vi "Set Internal Temp Limits.vi"(6 "parseError? T:Yes":bool=TRUE, 8 "error in (no error)":errorcluster, 9 "InternMin (-20.00 °C)":dbl=-20.0, 10 "InternMax (50.00 °C)":dbl=50.0, 11 "VISA resource name":refnum<visa-resource-name>) -> (0 "error out":errorcluster, 3 "VISA resource name out":refnum<visa-resource-name>)   [LabVIEW 2018, in "JULABO DeviceDriver.lvlib"]
doc: "This VI adjusts the upper and lower temperature limit for the internal temperature during external temperature control. <B>InternMax</B> and <B>InternMin</B> determine fixed limits for the temperature within the internal bath. The temperature controller cannot exceed these limits even if it would be necessary for achieving the temperature in an external system. Therefore it is possible that the external setpoint cannot be achieved.\n\nNote:\nThis function is not available for devices which do not have an external sensor plug. For these instruments the VI will return an error (-08 INVALID COMMAND)."
uses:
  JULABO DeviceDriver.lvlib
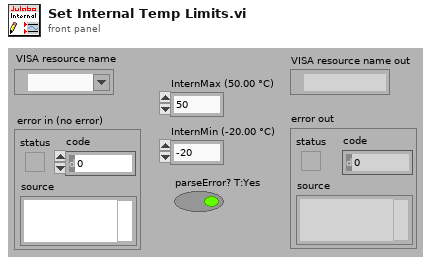
[diagram p1: front panel]
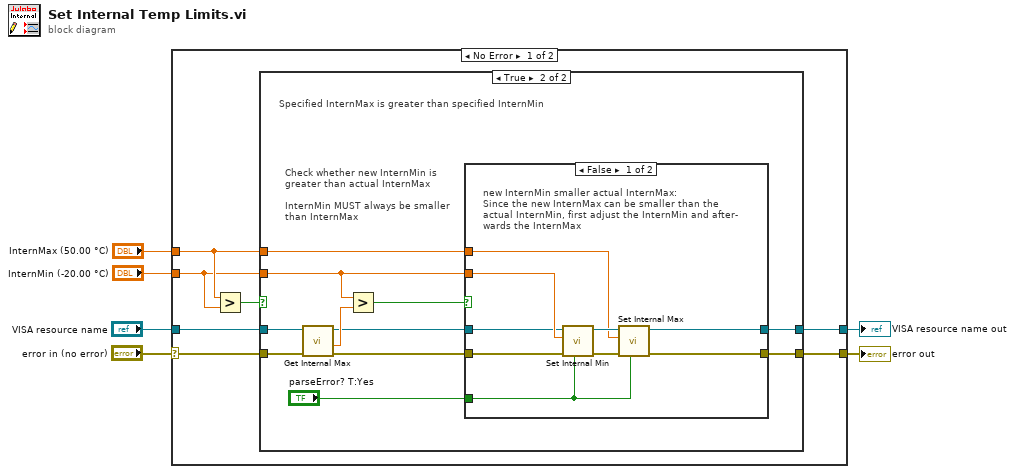
[diagram p0: block diagram]
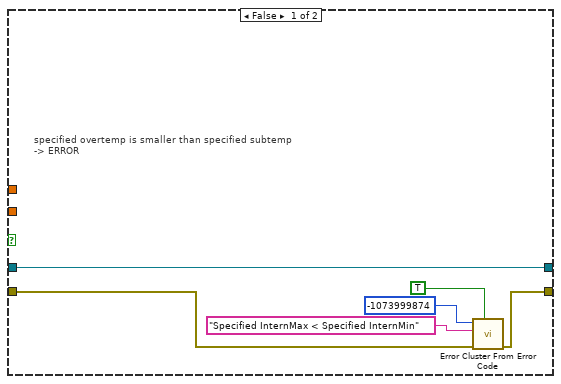
[diagram p2: hidden frame]
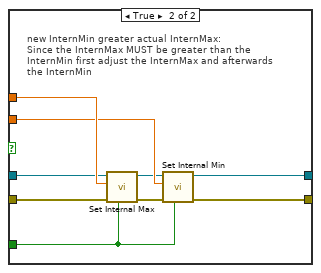
[diagram p3: hidden frame]
diagram:
  n1 = case shown="No Error" "error in (no error)" {
    selector: "error in (no error)" -> [w10 w49]
    tunnel: "VISA resource name" -> [w13 w50]
    tunnel: [w12 w50] -> w5
    tunnel: [w11 w49] -> w4
    tunnel: "InternMax (50.00 °C)" -> [w8 _]
    tunnel: "InternMin (-20.00 °C)" -> [w7 _]
    frame No Error {
      n2 = Greater?(x=w8, y=w7) -> (0:w9:bool)
      n3 = case shown="True" w9 {
        tunnel: w13 -> [w19 w26]
        tunnel: [w19 w29] -> w12
        tunnel: [w15 w28] -> w11
        tunnel: w10 -> [w14 w25]
        tunnel: w8 -> [_ w27]
        tunnel: w7 -> [_ w23]
        frame False {
          # "specified overtemp is smaller than specified subtemp\n-> ERROR"
          n4 = call <vilib>:"Error Cluster From Error Code.vi"("show call chain? (False)"=TRUE, "error in (no error)"=w14, "error message (\"\")"="Specified InternMax < Specified InternMin" ("error message (\"\")"), "error code (0)"=-1073999874) -> ("error out"=w15:errorcluster)  [unwired: 5 in]
        }
        frame True {
          # "Check whether new InternMin is\ngreater than actual InternMax\n\nInternMin MUST always be smaller\nthan InternMax"
          # "Specified InternMax is greater than specified InternMin"
          n5 = call "Get Internal Max.vi"("error in (no error)"=w25, "VISA resource name"=w26) -> ("error out"=w21:errorcluster, "IntMax (out)"=w24:dbl, "VISA resource name out"=w22:refnum<visa-resource-name>)  [unwired: 7 in]
          n6 = Greater?(x=w23, y=w24) -> (0:w20:bool)
          n7 = case shown="False" w20 {
            tunnel: "parseError? T:Yes" -> [w39 w48]
            tunnel: [w36 w41] -> w29
            tunnel: [w35 w40] -> w28
            tunnel: w27 -> [w34 w47]
            tunnel: w23 -> [w33 w46]
            tunnel: w22 -> [w32 w45]
            tunnel: w21 -> [w31 w44]
            frame False {
              # "new InternMin smaller actual InternMax:\nSince the new InternMax can be smaller than the \nactual InternMin, first adjust the InternMin and after-\nwards the InternMax"
              n8 = call "Set Internal Min.vi"("parseError? T:Yes"=w39, "error in (no error)"=w31, "InternMin (-20.00 °C)"=w33, "VISA resource name"=w32) -> ("error out"=w37:errorcluster, "VISA resource name out"=w38:refnum<visa-resource-name>)  [unwired: 6 in]
              n9 = call "Set Internal Max.vi"("parseError? T:Yes"=w39, "error in (no error)"=w37, "InternMax (50.00 °C)"=w34, "VISA resource name"=w38) -> ("error out"=w35:errorcluster, "VISA resource name out"=w36:refnum<visa-resource-name>)  [unwired: 6 in]
            }
            frame True {
              # "new InternMin greater actual InternMax:\nSince the InternMax MUST be greater than the\nInternMin first adjust the InternMax and afterwards \nthe InternMin"
              n10 = call "Set Internal Max.vi"("parseError? T:Yes"=w48, "error in (no error)"=w44, "InternMax (50.00 °C)"=w47, "VISA resource name"=w45) -> ("error out"=w42:errorcluster, "VISA resource name out"=w43:refnum<visa-resource-name>)  [unwired: 6 in]
              n11 = call "Set Internal Min.vi"("parseError? T:Yes"=w48, "error in (no error)"=w42, "InternMin (-20.00 °C)"=w46, "VISA resource name"=w43) -> ("error out"=w40:errorcluster, "VISA resource name out"=w41:refnum<visa-resource-name>)  [unwired: 6 in]
            }
          }
        }
      }
    }
    frame Error {
    }
  }
  "VISA resource name out" <- w5
  "error out" <- w4
